vi "Self Execution.vi"(6 "Any Data":variant, 8 "error in (no error)":errorcluster, 9 "Composite Task Group In":refnum<class "Composite Task Group.lvclass">, 10 "Message In":refnum<class "Message.lvclass">, 11 "Actor In":refnum<class "System Actor.lvclass">) -> (0 "error out":errorcluster, 1 "Composite Task Group Out":refnum<class "Composite Task Group.lvclass">, 2 "Message Out":refnum<class "Message.lvclass">)   [LabVIEW 2019, in "Composite Task Group.lvclass"]
uses:
  Composite Task Group.lvclass
  Actor/System Actor/System Actor.lvclass
  Message/Message.lvclass
  Composite Task Group.lvclass/Composite Task Group.ctl
  Messenger/Messenger/Messenger.lvclass
  Message/Type Def/CMD Type.ctl
  Message/Type Def/General CMD.ctl
  Message/Message.lvclass/Message.ctl
  Message/Public Data/Write CMD Type.vi
  Message/Public Data/Write General CMD.vi
  Message/Public Data/Write Single Task.vi
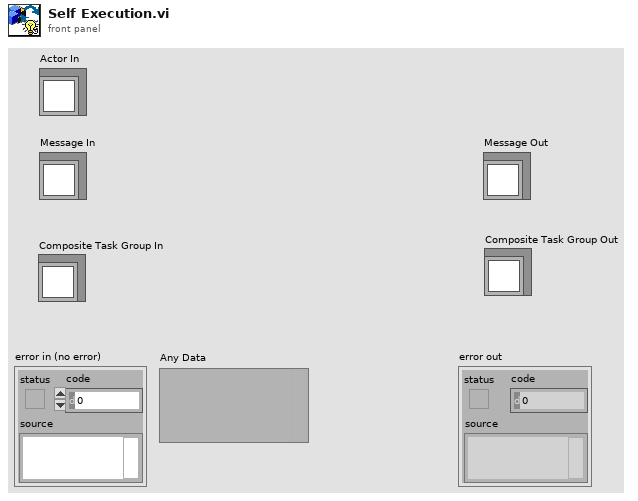
[diagram p1: front panel]
types:
  T1 = typedef "Next Task Unit.ctl" = cluster{"Next Task":refnum<class "Task Ancestor.lvclass">, "Mail To Next Actor":refnum<class "Mail Strategy.lvclass">, "Messenger Reference":refnum<data-value>}
  T2 = typedef "General CMD.ctl" = enum16{"None", "Stop", "Abort", "Running Task", "Running Batch Tasks", "Task Self Running", "Emergency Stop", "Subscribe", "UnSubscribe", "Pause"}
  T3 = typedef "CMD Type.ctl" = enum16{"None", "General CMD", "1st CMD", "2nd CMD", "3rd CMD", "4th CMD", "5th CMD", "6th CMD", "7th CMD"}
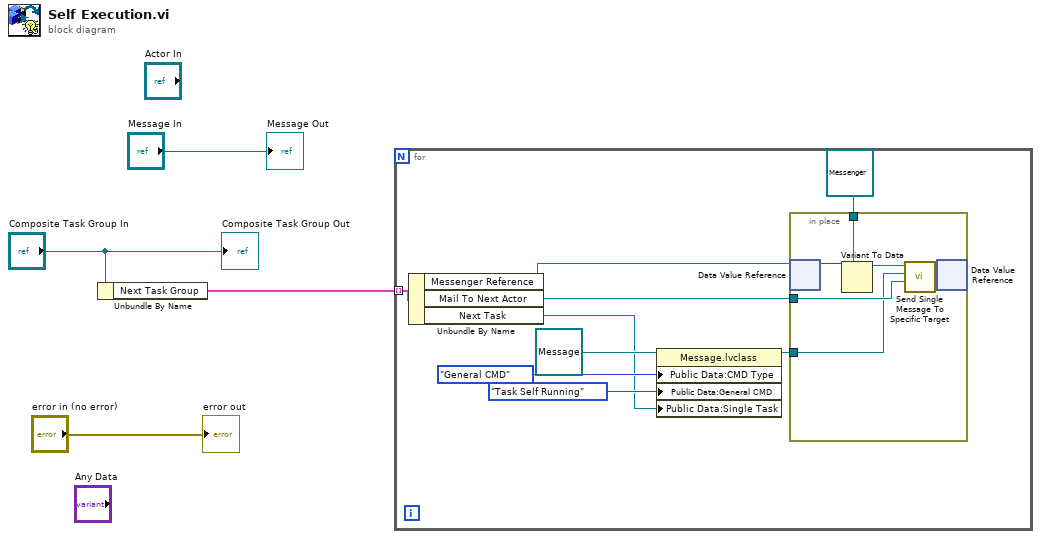
[diagram p0: block diagram]
diagram:
  n1 = Unbundle By Name("Composite Task Group In") -> ("Next Task Group"=w1:T1[])
  n2 = for {
    tunnel: w1 -> [w8] mode=indexing
    n3 = Unbundle By Name(w8) -> ("Messenger Reference"=w7:refnum<data-value>, "Mail To Next Actor"=w6:refnum<class "Mail Strategy.lvclass">, "Next Task"=w5:refnum<class "Task Ancestor.lvclass">)
    n4 = property class="Message.lvclass"(reference=refnum<class "Message.lvclass"> refnum ("Message.lvclass"), "Public Data:CMD Type"=CMD_Type."General CMD" ("CMD Type"), "Public Data:General CMD"=General_CMD."Task Self Running" ("General CMD"), "Public Data:Single Task"=w5) -> (reference out=w9:refnum<class "Message.lvclass">)  [unwired: 1 in, 1 out]
    n5 = in-place {
      in-place-border: w6 -> [w16]
      in-place-border: refnum<class "Messenger.lvclass"> refnum ("Messenger.lvclass") -> [w18]
      in-place-border: w9 -> [w14]
      n6 = in-place-dvr #1(w7) -> (w19:variant)  [unwired: 1 out]
      n7 = Variant To Data(type=w18, Variant=w19) -> (data=w17:refnum<class "Messenger.lvclass">)  [unwired: 1 in, 1 out]
      n8 = call-dynamic "Send Single Message To Specific Target.vi"("Mail Strategy In"=w16, "Message In"=w14, "Messenger in"=w17) -> ("Messenger out"=w15:refnum<class "Messenger.lvclass">)  [unwired: 7 in, 1 out]
      n9 = in-place-dvr #1(w15) -> ()  [unwired: 2 out]
    }
  }
  "error out" <- "error in (no error)"
  "Message Out" <- "Message In"
  "Composite Task Group Out" <- "Composite Task Group In"
